vi "sortMag (SubVI).vi"(11 "sortPhase":T2(array[cluster])) -> (3 "sortMag":T1(array[cluster]))   [LabVIEW 2011]
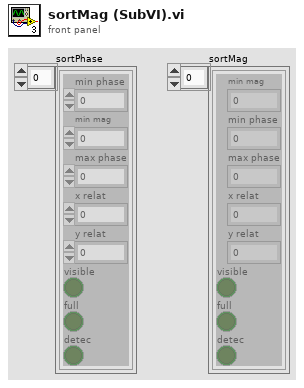
[diagram p1: front panel]
types:
  T1 = cluster{"min mag":dbl, "min phase":dbl, "max phase":dbl, "x relat":i32, "y relat":i32, "visible":bool, "full":bool, "detec":bool}[]
  T2 = cluster{"min phase":dbl, "min mag":dbl, "max phase":dbl, "x relat":i32, "y relat":i32, "visible":bool, "full":bool, "detec":bool}[]
  T3 = cluster{"min mag":dbl, "min phase":dbl, "max phase":dbl, "x relat":i32, "y relat":i32, "visible":bool, "full":bool, "detec":bool}
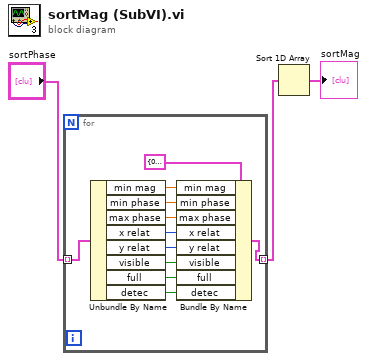
[diagram p0: block diagram]
diagram:
  n1 = for {
    tunnel: "sortPhase" -> [w14] mode=indexing
    tunnel: [w5] -> w1 mode=indexing
    n2 = Unbundle By Name(w14) -> ("min mag"=w13:dbl, "min phase"=w12:dbl, "max phase"=w11:dbl, "x relat"=w10:i32, "y relat"=w9:i32, "visible"=w8:bool, "full"=w7:bool, "detec"=w6:bool)
    n3 = Bundle By Name(cluster=T3 {"min mag"=0.0, "min phase"=0.0, "max phase"=0.0, "x relat"=0, "y relat"=0, "visible"=FALSE, "full"=FALSE, "detec"=FALSE} ("output cluster"), "min mag"=w13, "min phase"=w12, "max phase"=w11, "x relat"=w10, "y relat"=w9, "visible"=w8, "full"=w7, "detec"=w6) -> (w5:T3)
  }
  n4 = Sort 1D Array(array=w1) -> (sorted array=→"sortMag":T1)
